vi "All Discovered Nodes.vi"(8 "error in (no error)":errorcluster, 11 "DiscoveryService in":refnum<class "DiscoveryService.lvclass">) -> (0 "error out":errorcluster, 2 "Nodes":T1[](array[typedef]), 3 "DiscoveryService out":refnum<class "DiscoveryService.lvclass">)   [LabVIEW 2020, in "Vecto.lvlib" / "DiscoveryService.lvclass"]
uses:
  DiscoveryService.lvclass
  lv-volatus/messages/Discovery/Data.ctl
  lv-volatus/messages/Service/Data.ctl
  lv-volatus/messages/ServiceType/Enumeration.ctl
  DiscoveryService.lvclass/DiscoveryService.ctl
  lv-volatus/messages/ServiceType/ServiceType.lvlib
  lv-volatus/messages/Service/Service.lvlib
  lv-volatus/messages/Discovery/Discovery.lvlib
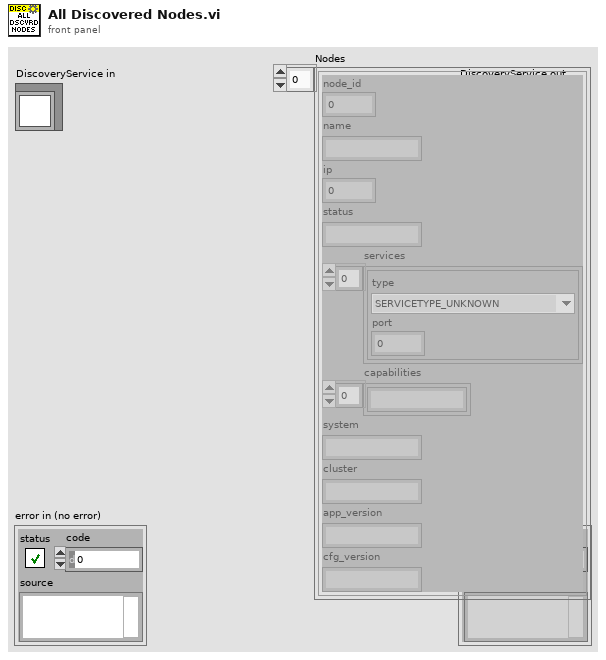
[diagram p1: front panel]
types:
  T1 = typedef "Discovery.lvlib/Data.ctl" = cluster{"node_id":u32, "name":string, "ip":u32, "status":string, "services":T2[], "capabilities":string[], "system":string, "cluster":string, "app_version":string, "cfg_version":string}
  T2 = typedef "Service.lvlib/Data.ctl" = cluster{"type":T3, "port":i32}
  T3 = typedef "ServiceType.lvlib/Enumeration.ctl" = enum16{"SERVICETYPE_UNKNOWN", "SERVICETYPE_TCPSERVER", "SERVICETYPE_HTTPSERVER"}
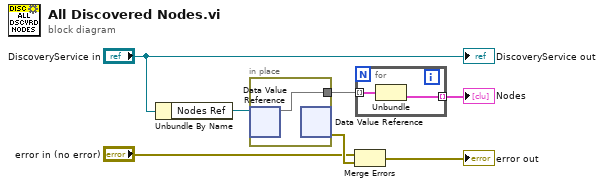
[diagram p0: block diagram]
diagram:
  n1 = Unbundle By Name("DiscoveryService in") -> ("Nodes Ref"=w7:refnum<data-value>)
  n2 = in-place {
    in-place-border: [w8] -> w3
    n3 = in-place-dvr #1(w7) -> (w8:map{u32, T1})  [unwired: 1 out]
    n4 = in-place-dvr #1() -> (w6:errorcluster)  [unwired: 1 in, 1 out]
  }
  n5 = Merge Errors("error in (no error)", w6) -> (→"error out":errorcluster)
  n6 = for {
    tunnel: w3 -> [w10] mode=indexing
    tunnel: [w9] -> w2 mode=indexing
    n7 = Unbundle(w10) -> ("Discovery"=w9:T1)  [unwired: 1 out]
  }
  "Nodes" <- w2
  "DiscoveryService out" <- "DiscoveryService in"
